vi "Read (Single Point).vi"(8 "error in (no error)":errorcluster, 9 "Ring":u16(ring) items=["CH2"=2, "CH1"=1], 10 "Combo Box":string(combo)="VOLT", 11 "VISA resource name":refnum<visa-resource-name>) -> (0 "error out":errorcluster, 2 "Measurement":dbl, 3 "VISA resource name out":refnum<visa-resource-name>)   [LabVIEW 2024, in "EFmeter.lvlib"]
doc: "Reads and returns a single measurement from the instrument."
uses:
  <instrlib>/EFmeter/EFmeter.lvlib
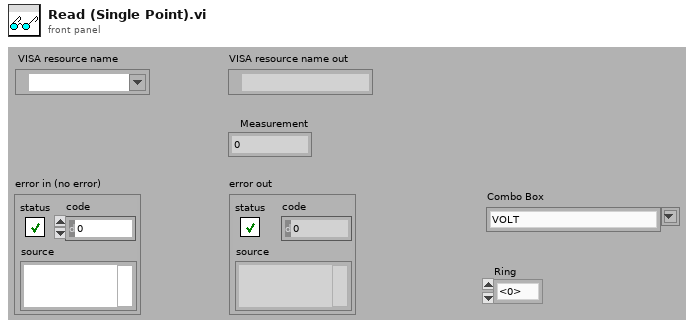
[diagram p1: front panel]
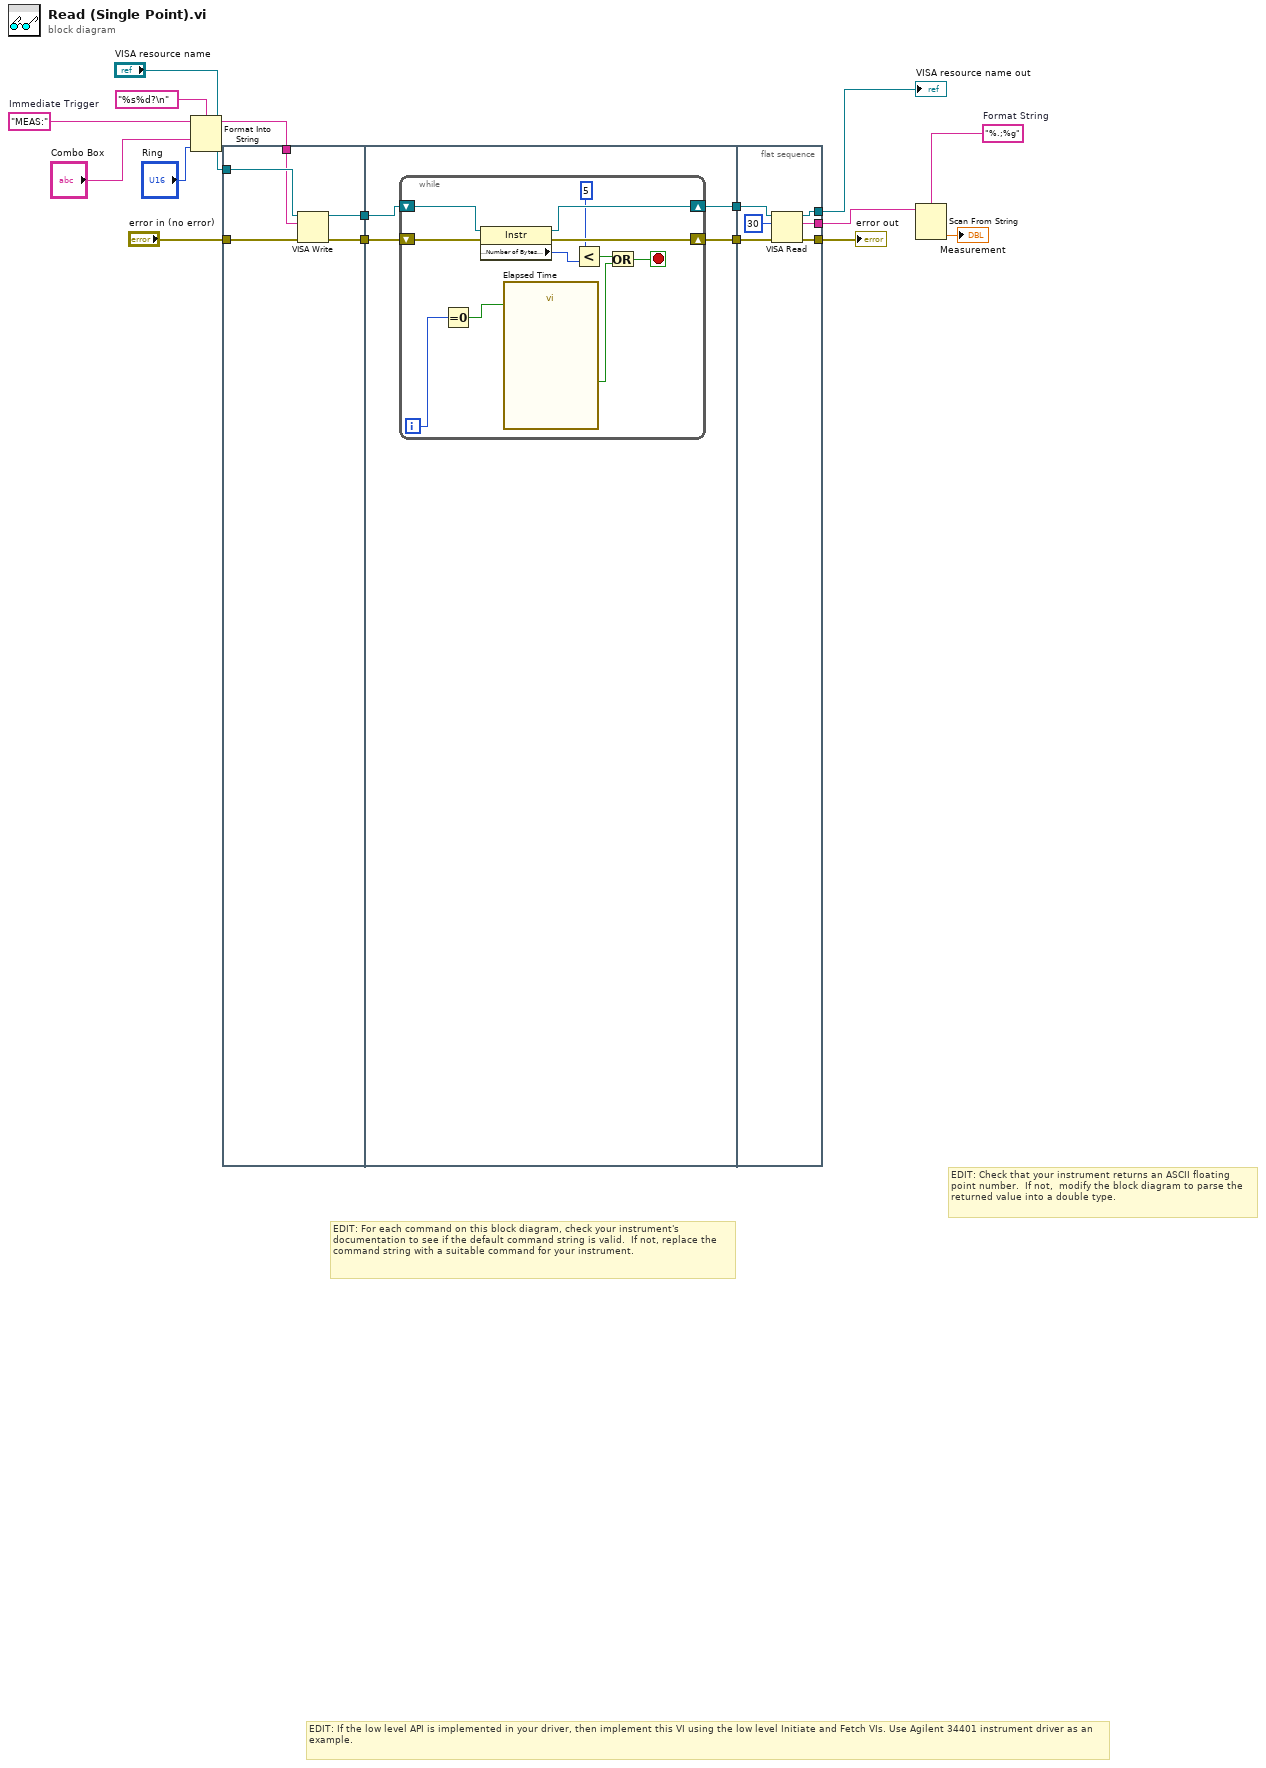
[diagram p0: block diagram]
diagram:
  w13 = "MEAS:"  # Immediate Trigger
  w16 = "%.;%g"  # Format String
  # "EDIT: If the low level API is implemented in your driver, then implement this VI using the low level Initiate and Fetch VIs. Use Agilent 34401 instrument driver as an example."
  # "EDIT: Check that your instrument returns an ASCII floating point number.  If not,  modify the block diagram to parse the returned value into a double type."
  # "EDIT: For each command on this block diagram, check your instrument's documentation to see if the default command string is valid.  If not, replace the command string with a suitable command for your instrument."
  n1 = Format Into String(format string="%s%d?\n", initial string=w13, "Combo Box", "Ring") -> (resulting string=w1:string)  [unwired: 1 in, 1 out]
  n2 = flat-sequence {
    tunnel: [w19] -> w10
    tunnel: [w18] -> w9
    tunnel: "error in (no error)" -> [w21]
    tunnel: "VISA resource name" -> [w20]
    tunnel: w1 -> [w17]
    tunnel: w10 -> [w24]
    tunnel: w9 -> [w25]
    tunnel: [w22] -> w8
    tunnel: [w23] -> w2
    tunnel: w8 -> [w42]
    tunnel: [w41] -> w7
    tunnel: [w40] -> w6
    tunnel: [w39] -> w5
    tunnel: w2 -> [w38]
    frame #0 {
      n3 = VISA Write(VISA resource name=w20, write buffer=w17, error in (no error)=w21) -> (VISA resource name out=w18:refnum<visa-resource-name>, error out=w19:errorcluster)  [unwired: 1 out]
    }
    frame #1 {
      n4 = while {
        shift-right: [w31] -> w22
        shift-left: w24 -> [w33]
        shift-right: [w32] -> w23
        shift-left: w25 -> [w34]
        i -> [w29]
        stop <- w35 stop-if-true
        n5 = Equal To 0?(x=w29) -> (x = 0?=w30:bool)
        n6 = property class="Instr"(reference=w34, error in=w33) -> (reference out=w32:refnum<visa-resource-name>, error out=w31:errorcluster, "Serial Settings:Number of Bytes at Serial Port"=w28:u32)
        n7 = call "Elapsed Time"("Reset"=w30) -> ("Time has Elapsed"=w36:bool)  [unwired: 11 in, 7 out]
        n8 = Less?(x=u32 5, y=w28) -> (x < y?=w26:bool)
        n9 = Or(x=w26, y=w36) -> (x .or. y?=w35:bool)
      }
    }
    frame #2 {
      n10 = VISA Read(VISA resource name=w38, byte count=u32 30, error in (no error)=w42) -> (VISA resource name out=w39:refnum<visa-resource-name>, read buffer=w40:string, error out=w41:errorcluster)  [unwired: 1 out]
    }
  }
  n11 = Scan From String(format string=w16, input string=w6) -> (output 1=→"Measurement":dbl)  [unwired: 3 in, 3 out]
  "error out" <- w7
  "VISA resource name out" <- w5
